vi "Logging Message Loop.vi"(8 "error in (no error)":errorcluster, 10 "Data Queue":refnum<queue>, 11 "Message Queues":T1) -> (0 "error out":errorcluster)   [LabVIEW 2018, in "Logging.lvlib"]
doc: "The message loop subVI to handle messages pertaining to logging data."
uses:
  Logging.lvlib
  support/Message Queue/All Message Queues.ctl
  support/Message Queue/Message Cluster.ctl
  Logging Configuration.ctl
  Logging State.ctl
  support/Message Queue/Enqueue Message (Single).vi
  <vilib>/Utility/error.llb/Error Cluster From Error Code.vi
  <vilib>/ErrorRing/Error Ring.xnode
  support/Message Queue/Message Queue.lvlib
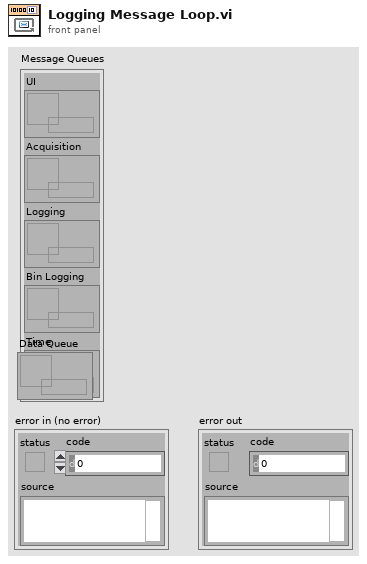
[diagram p1: front panel]
types:
  T1 = typedef "Message Queue.lvlib/All Message Queues.ctl" = cluster{"UI":refnum<queue>, "Acquisition":refnum<queue>, "Logging":refnum<queue>, "Bin Logging":refnum<queue>, "Time":refnum<queue>}
  T2 = typedef "Logging.lvlib/Logging Configuration.ctl" = cluster{"Log File Base Path":path, "TDMS File Reference":refnum<k34>, "Log File Offsite Path":path, "Project code":string, "Bin File Reference":refnum<k34>}
  T3 = typedef "Logging.lvlib/Logging State.ctl" = enum16{"Idle", "Logging"}
  T4 = enum16{"open", "open or create", "create or replace", "create", "open (read-only)"}
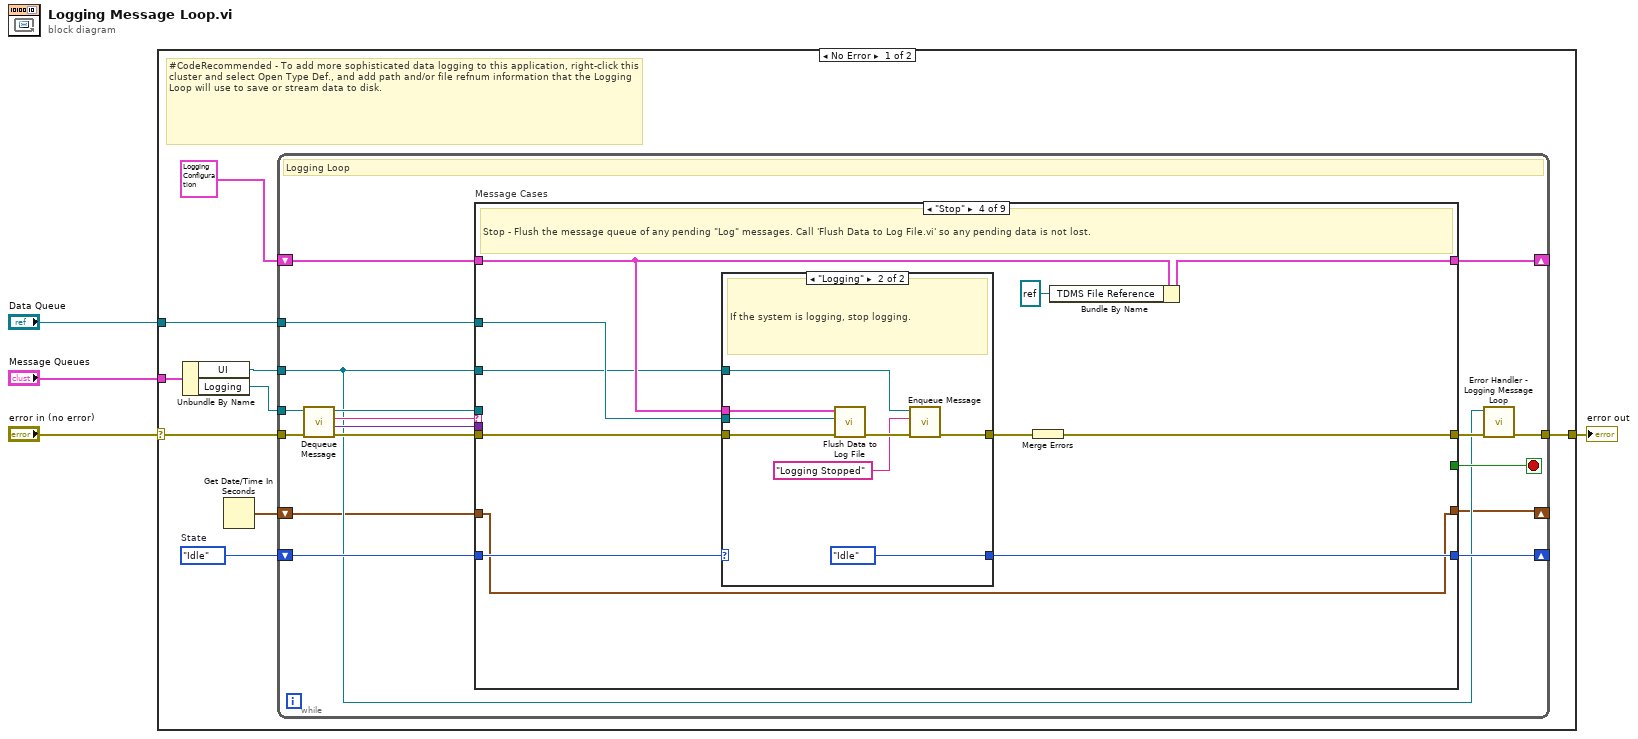
[diagram p0: block diagram]
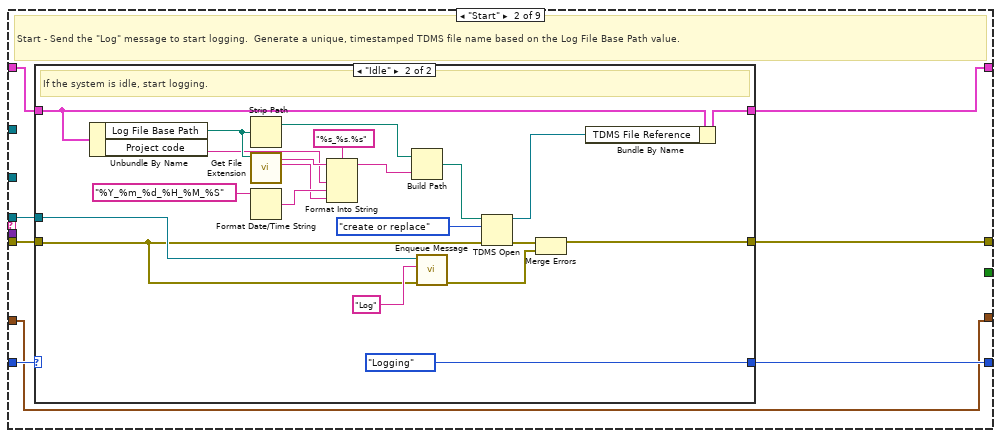
[diagram p3: hidden frame]
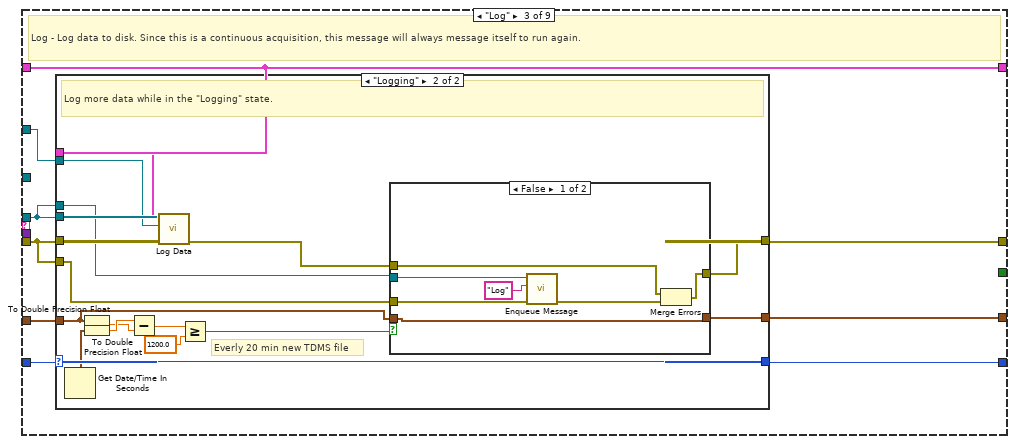
[diagram p5: hidden frame]
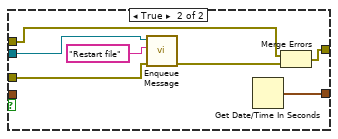
[diagram p7: hidden frame]
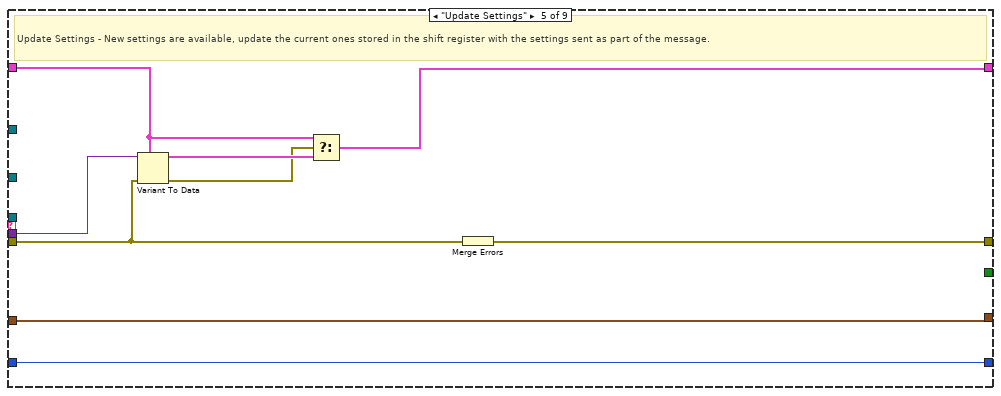
[diagram p9: hidden frame]
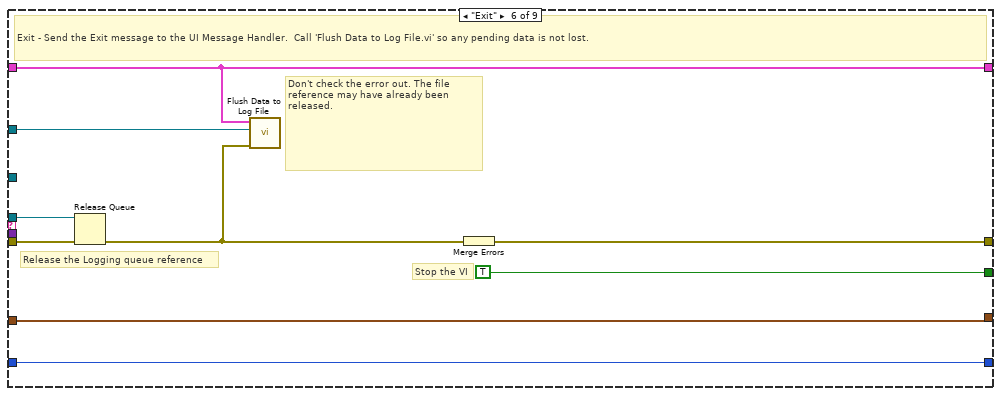
[diagram p10: hidden frame]
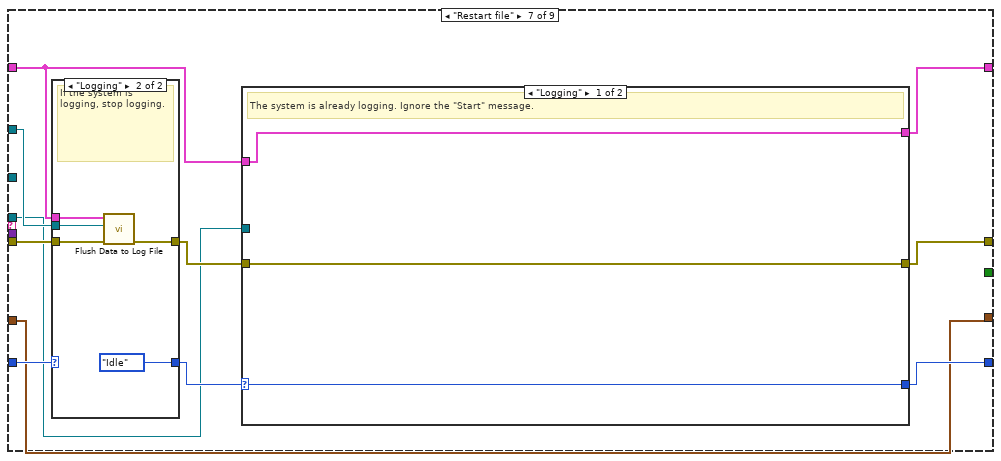
[diagram p11: hidden frame]
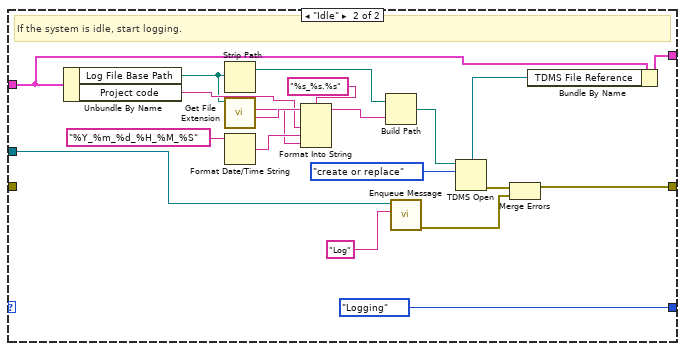
[diagram p12: hidden frame]
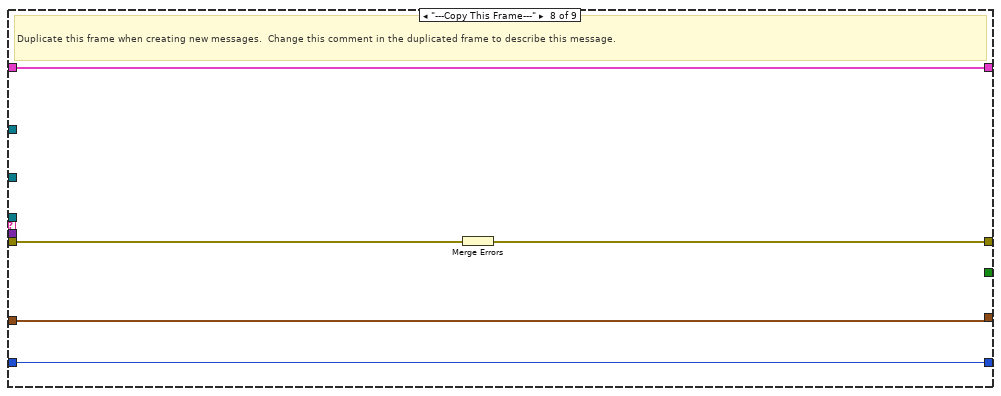
[diagram p14: hidden frame]
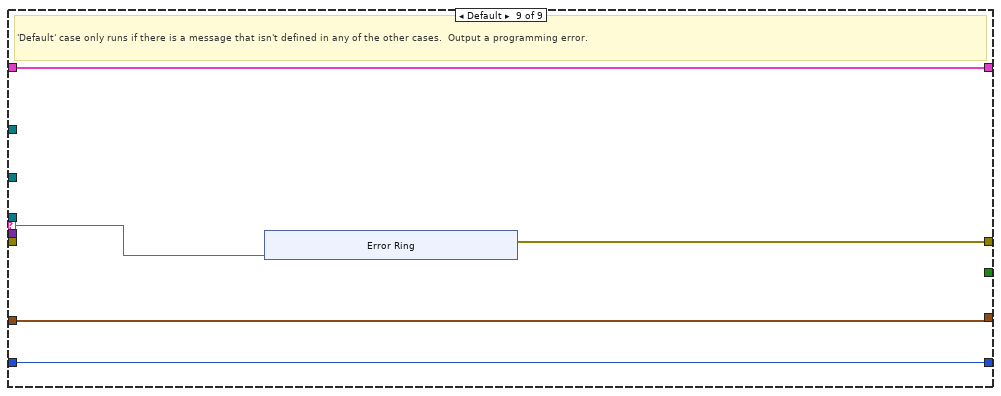
[diagram p15: hidden frame]
diagram:
  n1 = case shown="No Error" "error in (no error)" {
    selector: "error in (no error)" -> [w9 w206]
    tunnel: "Message Queues" -> [w13 _]
    tunnel: [w11 w206] -> w3
    tunnel: "Data Queue" -> [w8 _]
    frame No Error {
      w6 = Logging_State."Idle"  # State
      # "#CodeRecommended - To add more sophisticated data logging to this application, right-click this cluster and select Open Type Def., and add path and/or file refnum information that the Logging Loop will use to save or stream data to disk."
      n2 = Unbundle By Name(w13) -> ("UI"=w7:refnum<queue>, "Logging"=w12:refnum<queue>)
      n3 = Get Date/Time In Seconds() -> (seconds since 1Jan1904=w5:timestamp)
      n4 = while {
        tunnel: w12 -> [w22]
        shift-right: [w29] -> _
        shift-left: T2 {"Log File Base Path"=path "", "TDMS File Reference"=refnum, "Log File Offsite Path"=path "", "Project code"="", "Bin File Reference"=refnum} ("Logging Configuration") -> [w30]
        tunnel: w7 -> [w16]
        tunnel: w8 -> [w21]
        shift-right: [w19] -> _
        shift-left: w6 -> [w20]
        tunnel: w9 -> [w27]
        tunnel: [w18] -> w11
        shift-right: [w14] -> _
        shift-left: w5 -> [w15]
        stop <- w28 stop-if-true
        # "Logging Loop"
        n5 = call "Dequeue Message.vi"("error in (no error)"=w27, "Message Queue"=w22) -> ("error out"=w26:errorcluster, "Message Data"=w24:variant, "Message"=w25:string, "dup Message Queue"=w23:refnum<queue>)  [unwired: 6 in]
        n6 = case "Message Cases" shown="\"Stop\"" w25 {
          selector: w25 -> [_ _ _ _ _ _ _ _ w195]
          tunnel: w23 -> [_ w41 w70 _ _ w144 w150 _ _]
          tunnel: w26 -> [w33 w40 w71 w113 w132 w145 w157 w193 _]
          tunnel: [w33 w42 w75 w119 w138 w146 w153 w191 w196] -> w17
          tunnel: w30 -> [w34 w39 w74 w114 w136 w142 w155 w192 w198]
          tunnel: [w34 w38 w74 w117 w133 w142 w152 w192 w198] -> w29
          tunnel: [_ _ _ _ _ TRUE _ _ _] -> w28
          tunnel: w24 -> [_ _ _ _ w137 _ _ _ _]
          tunnel: w16 -> [_ _ _ w110 _ _ _ _ _]
          tunnel: w21 -> [_ _ w69 w115 _ w141 w156 _ _]
          tunnel: w20 -> [w32 w37 w73 w112 w131 w140 w158 w190 w197]
          tunnel: [w32 w36 w72 w111 w131 w140 w149 w190 w197] -> w19
          tunnel: w15 -> [w31 w35 w68 w109 w130 w139 w148 w189 w194]
          tunnel: [w31 w35 w67 w109 w130 w139 w148 w189 w194] -> w14
          frame "Initialize" {
            # "Initialize - gets called when first launched. Currently a no-op."
          }
          frame "Start" {
            # "Start - Send the \"Log\" message to start logging.  Generate a unique, timestamped TDMS file name based on the Log File Base Path value."
            n7 = case shown="\"Idle\"" w37 {
              selector: w37 -> [w44 _]
              tunnel: [w43 w48] -> w42
              tunnel: w41 -> [_ w49]
              tunnel: w40 -> [w43 w47]
              tunnel: w39 -> [w45 w50]
              tunnel: [w45 w52] -> w38
              tunnel: [w44 Logging_State."Logging" ("State")] -> w36
              frame "Logging" {
                # "The system is already logging. Ignore the \"Start\" message."
              }
              frame "Idle" {
                # "If the system is idle, start logging."
                n8 = Unbundle By Name(w50) -> ("Log File Base Path"=w65:path, "Project code"=w46:string)
                n9 = Strip Path(path=w65) -> (stripped path=w62:path)  [unwired: 1 out]
                n10 = call <vilib>:"Get File Extension.vi"("file"=w65) -> ("filename without extension"=w63:string, "lowercase file extension"=w59:string)  [unwired: 6 in, 3 out]
                n11 = Format Date/Time String(time format string (%c)="%Y_%m_%d_%H_%M_%S") -> (date/time string=w60:string)  [unwired: 2 in]
                n12 = Format Into String(format string="%s_%s.%s", initial string=w63, w46, w60, w59) -> (resulting string=w58:string)  [unwired: 1 in, 1 out]
                n13 = Build Path(base path=w62, name or relative path=w58) -> (appended path=w57:path)
                n14 = call-poly "Enqueue Message.vi"("error in (no error)"=w47, "Message"="Log", "Message Queue"=w49) -> ("error out"=w55:errorcluster)  [unwired: 7 in, 1 out]
                n15 = TDMS Open(8:w47, 10:T4."create or replace" ("operation (0:open)"), 11:w57) -> (0:w56:errorcluster, 3:w53:refnum<k34>)  [unwired: 4 in]
                n16 = Merge Errors(w56, w55) -> (w48:errorcluster)
                n17 = Bundle By Name(cluster=w50, "TDMS File Reference"=w53) -> (w52:T2)
              }
            }
          }
          frame "Log" {
            # "Log - Log data to disk. Since this is a continuous acquisition, this message will always message itself to run again."
            n18 = case shown="\"Logging\"" w73 {
              selector: w73 -> [w78 w94]
              tunnel: [w77 w90] -> w75
              tunnel: w70 -> [_ _]
              tunnel: w69 -> [_ w88]
              tunnel: w71 -> [w77 w93]
              tunnel: w74 -> [_ w87]
              tunnel: [w78 w94] -> w72
              tunnel: w71 -> [_ w92]
              tunnel: w70 -> [_ w89]
              tunnel: w68 -> [w76 w81]
              tunnel: [w76 w82] -> w67
              frame "Idle" {
                # "Ignore \"Log\" messages when the logging is idle."
              }
              frame "Logging" {
                # "Everly 20 min new TDMS file"
                # "Log more data while in the \"Logging\" state."
                n19 = Get Date/Time In Seconds() -> (seconds since 1Jan1904=w86:timestamp)
                n20 = To Double Precision Float(number=w81) -> (double precision float=w79:dbl)
                n21 = To Double Precision Float(number=w86) -> (double precision float=w80:dbl)
                n22 = Subtract(x=w80, y=w79) -> (x-y=w85:dbl)
                n23 = call "Log Data.vi"("error in (no error)"=w93, "Data Queue"=w88, "Logging Configuration"=w87) -> ("error out"=w91:errorcluster)  [unwired: 8 in]
                n24 = Greater Or Equal?(x=w85, y=1200.0) -> (x >= y?=w83:bool)
                n25 = case shown="False" w83 {
                  tunnel: w92 -> [w100 w105]
                  tunnel: w89 -> [w98 w106]
                  tunnel: w91 -> [w97 w104]
                  tunnel: [w96 w103] -> w90
                  tunnel: [w95 w102] -> w82
                  tunnel: w81 -> [w95 _]
                  frame False {
                    n26 = call-poly "Enqueue Message.vi"("error in (no error)"=w100, "Message"="Log", "Message Queue"=w98) -> ("error out"=w101:errorcluster)  [unwired: 7 in, 1 out]
                    n27 = Merge Errors(w97, w101) -> (w96:errorcluster)
                  }
                  frame True {
                    n28 = call-poly "Enqueue Message.vi"("error in (no error)"=w105, "Message"="Restart file", "Message Queue"=w106) -> ("error out"=w108:errorcluster)  [unwired: 7 in, 1 out]
                    n29 = Get Date/Time In Seconds() -> (seconds since 1Jan1904=w102:timestamp)
                    n30 = Merge Errors(w104, w108) -> (w103:errorcluster)
                  }
                }
              }
            }
          }
          frame "Stop" {
            # "Stop - Flush the message queue of any pending \"Log\" messages. Call 'Flush Data to Log File.vi' so any pending data is not lost."
            n31 = case shown="\"Logging\"" w112 {
              selector: w112 -> [w120 _]
              tunnel: [w121 w124] -> w118
              tunnel: w115 -> [_ w128]
              tunnel: w114 -> [_ w127]
              tunnel: w113 -> [w121 w126]
              tunnel: [w120 Logging_State."Idle" ("State")] -> w111
              tunnel: w110 -> [_ w123]
              frame "Idle" {
                # "The system is already idle. Ignore the \"Stop\" message."
              }
              frame "Logging" {
                # "If the system is logging, stop logging."
                n32 = call "Flush Data to Log File.vi"("error in (no error)"=w126, "Data Queue"=w128, "Logging Configuration"=w127) -> ("error out"=w129:errorcluster)  [unwired: 8 in]
                n33 = call-poly "Enqueue Message.vi"("error in (no error)"=w129, "Message"="Logging Stopped", "Message Queue"=w123) -> ("error out"=w124:errorcluster)  [unwired: 7 in, 1 out]
              }
            }
            n34 = Merge Errors(w118) -> (w119:errorcluster)
            n35 = Bundle By Name(cluster=w114, "TDMS File Reference"=refnum<k34> refnum) -> (w117:T2)
          }
          frame "Update Settings" {
            # "Update Settings - New settings are available, update the current ones stored in the shift register with the settings sent as part of the message."
            n36 = Variant To Data(error in=w132, type=w136, Variant=w137) -> (data=w135:T2, error out=w134:errorcluster)
            n37 = Select(t=w136, s=w134, f=w135) -> (s? t:f=w133:T2)
            n38 = Merge Errors(w132) -> (w138:errorcluster)
          }
          frame "Exit" {
            # "Don't check the error out. The file reference may have already been released."
            # "Release the Logging queue reference"
            # "Stop the VI"
            # "Exit - Send the Exit message to the UI Message Handler.  Call 'Flush Data to Log File.vi' so any pending data is not lost."
            n39 = Release Queue(queue=w144, error in (no error)=w145) -> (error out=w143:errorcluster)  [unwired: 1 in, 2 out]
            n40 = call "Flush Data to Log File.vi"("error in (no error)"=w143, "Data Queue"=w141, "Logging Configuration"=w142) -> ()  [unwired: 8 in, 1 out]
            n41 = Merge Errors(w143) -> (w146:errorcluster)
          }
          frame "Restart file" {
            n42 = case shown="\"Logging\"" w158 {
              selector: w158 -> [w182 _]
              tunnel: [w183 w184] -> w151
              tunnel: w156 -> [_ w188]
              tunnel: w155 -> [_ w187]
              tunnel: w157 -> [w183 w186]
              tunnel: [w182 Logging_State."Idle" ("State")] -> w154
              frame "Idle" {
                # "The system is already idle. Ignore the \"Stop\" message."
              }
              frame "Logging" {
                # "If the system is logging, stop logging."
                n43 = call "Flush Data to Log File.vi"("error in (no error)"=w186, "Data Queue"=w188, "Logging Configuration"=w187) -> ("error out"=w184:errorcluster)  [unwired: 8 in]
              }
            }
            n44 = case shown="\"Logging\"" w154 {
              selector: w154 -> [w161 _]
              tunnel: [w159 w166] -> w153
              tunnel: [w160 w168] -> w152
              tunnel: [w161 Logging_State."Logging" ("State")] -> w149
              tunnel: w155 -> [w160 w164]
              tunnel: w151 -> [w159 _]
              tunnel: w150 -> [_ w162]
              frame "Logging" {
                # "The system is already logging. Ignore the \"Start\" message."
              }
              frame "Idle" {
                # "If the system is idle, start logging."
                n45 = Unbundle By Name(w164) -> ("Log File Base Path"=w163:path, "Project code"=w165:string)
                n46 = Strip Path(path=w163) -> (stripped path=w178:path)  [unwired: 1 out]
                n47 = call <vilib>:"Get File Extension.vi"("file"=w163) -> ("filename without extension"=w179:string, "lowercase file extension"=w175:string)  [unwired: 6 in, 3 out]
                n48 = Format Date/Time String(time format string (%c)="%Y_%m_%d_%H_%M_%S") -> (date/time string=w176:string)  [unwired: 2 in]
                n49 = Format Into String(format string="%s_%s.%s", initial string=w179, w165, w176, w175) -> (resulting string=w174:string)  [unwired: 1 in, 1 out]
                n50 = Build Path(base path=w178, name or relative path=w174) -> (appended path=w173:path)
                n51 = call-poly "Enqueue Message.vi"("Message"="Log", "Message Queue"=w162) -> ("error out"=w171:errorcluster)  [unwired: 8 in, 1 out]
                n52 = TDMS Open(10:T4."create or replace" ("operation (0:open)"), 11:w173) -> (0:w172:errorcluster, 3:w169:refnum<k34>)  [unwired: 5 in]
                n53 = Merge Errors(w172, w171) -> (w166:errorcluster)
                n54 = Bundle By Name(cluster=w164, "TDMS File Reference"=w169) -> (w168:T2)
              }
            }
          }
          frame "---Copy This Frame---" {
            # "Duplicate this frame when creating new messages.  Change this comment in the duplicated frame to describe this message."
            n55 = Merge Errors(w193) -> (w191:errorcluster)
          }
          frame Default {
            # "'Default' case only runs if there is a message that isn't defined in any of the other cases.  Output a programming error."
            n56 = xnode "Error Ring"("parameter 0"=w195) -> ("error out"=w196:errorcluster)
          }
        }
        n57 = call "Error Handler - Logging Message Loop.vi"("error in (no error)"=w17, "Message Queue"=w16) -> ("dup error in"=w18:errorcluster)  [unwired: 8 in, 1 out]
      }
    }
    frame Error {
    }
  }
  "error out" <- w3
